vi "Open Log.vi"(8 "error in (no error)":errorcluster, 11 "Message Queue":refnum<queue>) -> (0 "error out":errorcluster)   [LabVIEW 2014, in "Logger.lvlib"]
uses:
  Logger.lvlib
  support/Message Queue/Message Queue.lvlib
  support/Message Queue/Message Cluster.ctl
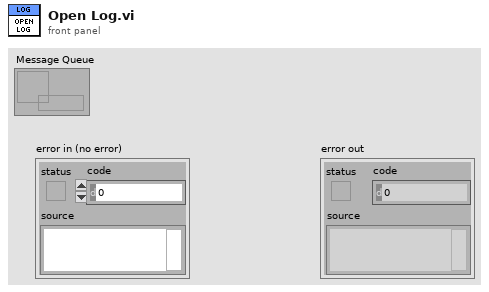
[diagram p1: front panel]
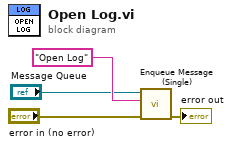
[diagram p0: block diagram]
diagram:
  n1 = call "Enqueue Message (Single).vi"("error in (no error)"="error in (no error)", "Message"="Open Log", "Message Queue"="Message Queue") -> ("error out"=→"error out":errorcluster)  [unwired: 7 in, 1 out]
